vi "MAIN_TUBES_ANGGUN.vi"() -> ()   [LabVIEW 2025]
uses:
  <vilib>/addons/database/Connection.llb/DB Tools Open Connec (Path).vi
  <vilib>/Instr/_visa.llb/VISA Configure Serial Port (Instr).vi
  <vilib>/addons/database/Auxilliary.llb/DB Tools Format Datetime String (Time Stamp).vi
  <vilib>/addons/database/NI_Database_API.lvlib
panel:
  out "Time Stamp Indicator - Tall 5":timestamp format="%<%.0X\n%x>T"
  out "concatenated string":string
  out "Hasil Query 3":string
  out "error out 6":errorcluster
  out "Hasil Query 2":string
  out "concatenated string 2":string
  out "DatabaseSensor":bool
  out "error out 5":errorcluster
  in  "error in":errorcluster
  out "Ultra":string
  out "error out 4":errorcluster
  out "element":string
  out "Numeric":i32
  out "x+y":i32
  out "index of element":i32
  out "s? t:f":i32
  out "output array":string[](array[string])
  out "Array identitas":string[][](array[string])
  out "status Sistem":bool
  out "Hasil Query":string
  in  "error in (no error) 6":errorcluster
  out "error in (no error) 5":errorcluster
  out "Datetime":string
  in  "baud rate (9600)":u32=115200
  out "Com":string
  out "Pressure":string
  out "Suhu":string
  out "Serial Settings:Number of Bytes at Serial Port":u32
  out "Kemiringan":string
  out "Relay":string
  out "Motor":string
  in  "Tab Control 2":enum32{"Page 1"}(tab)
  out "Cancel":bool
  out "error out 2":errorcluster
  out "Hardware and Database":bool
  out "Login by":string
  out "Cancel 2":bool
  out "error out 3":errorcluster
  in  "error in (no error)":errorcluster
  in  "error in (no error) 2":errorcluster
  in  "error in (no error) 3":errorcluster
  out "Array tables":string[][](array[string])
  in  "error in (no error) 4":errorcluster
  out "error out":errorcluster
  in  "Tab Control":T1(tab)
  out "Role":string
  out "Time Stamp Indicator - Tall":timestamp format="%<%.0X\n%x>T"
  in  "Database":bool
  in  "Sign Up":bool
  in  "Log Out Square":bool
  in  "Graph Button":bool
  out "SERVO":bool
  out "POMPA":bool
  out "GRAFIK SENSOR ULTRASONIC":waveform(dbl)(graph) caption="Waveform Chart - Dark"
  out "MOTOR 2":bool
  out "INFRARED 2":bool
  out "MAX":bool
  out "MIN":bool
  out "WATER LEVEL TANK 2":dbl(slide) scale=0.0..10.0
  out "Time Stamp Indicator - Tall 3":timestamp format="%<%.0X\n%x>T"
  in  "Tab Setting":enum32{"Page 1"}(tab)
  out "read buffer":string
  in  "Nilai":string(combo)
  in  "Pilihan Sensor & Aktuator":string(combo)
  in  "Settings Button":bool
  in  "write buffer":string
  in  "Delay":string
  in  "Database  2":bool
  in  "Home Button":bool
  out "Pompa":string
  out "Motor 2":string
  out "Infra":string
  out "GRAFIK SENSOR INFRARED":waveform(i32)(graph) caption="Waveform Chart - Dark"
  out "Servo":string
  in  "Refresh Square":bool
  in  "Combo Box - Autocomplete":string(combo)
  in  "Combo Box - Dropdown 2":string(combo)
  in  "Search Button":bool
  in  "Database Sensor":bool
  in  "TABEL DATA USER":i32(listbox)
  in  "Home Button 2":bool
  in  "Graph Button 2":bool
  in  "connection information":path=path "D:/TUBES_SCADA_FIX/database.udl"
  out "Time Stamp Indicator - Tall 2":timestamp format="%<%.0X\n%x>T"
  in  "ATUR WAKTU":timestamp format="%<%.0X %x>T"
  in  "Combo Box - Dropdown 3":string(combo)
  in  "Combo Box - Autocomplete 2":string(combo)
  in  "Refresh Square 2":bool
  in  "Search Button 2":bool
  out "Time Stamp Indicator - Tall 4":timestamp format="%<%.0X\n%x>T"
  in  "Database User":bool
  in  "TABEL DATA SENSOR":i32(listbox)
  in  "Home Button 3":bool
  in  "Graph Button 3":bool
  # "(231, 230, 230)"
  # "RANCANG BANGUN MONITORING  FILLING MACHINE WITH LABVIEW"
  # "GRAFIK SENSOR ULTRASONIC"
  # "CM"
  # "GRAFIK SENSOR INFRARED"
  # "Jumlah Pembacaan Sensor &"
  # "Aksi Aktuator (Hidup/Mati)"
  # "Waktu Delay Setiap Pembacaan"
  # "MENCARI DATA USER"
  # "Refresh"
  # "MENCARI DATA SENSOR"
  # "Refresh"
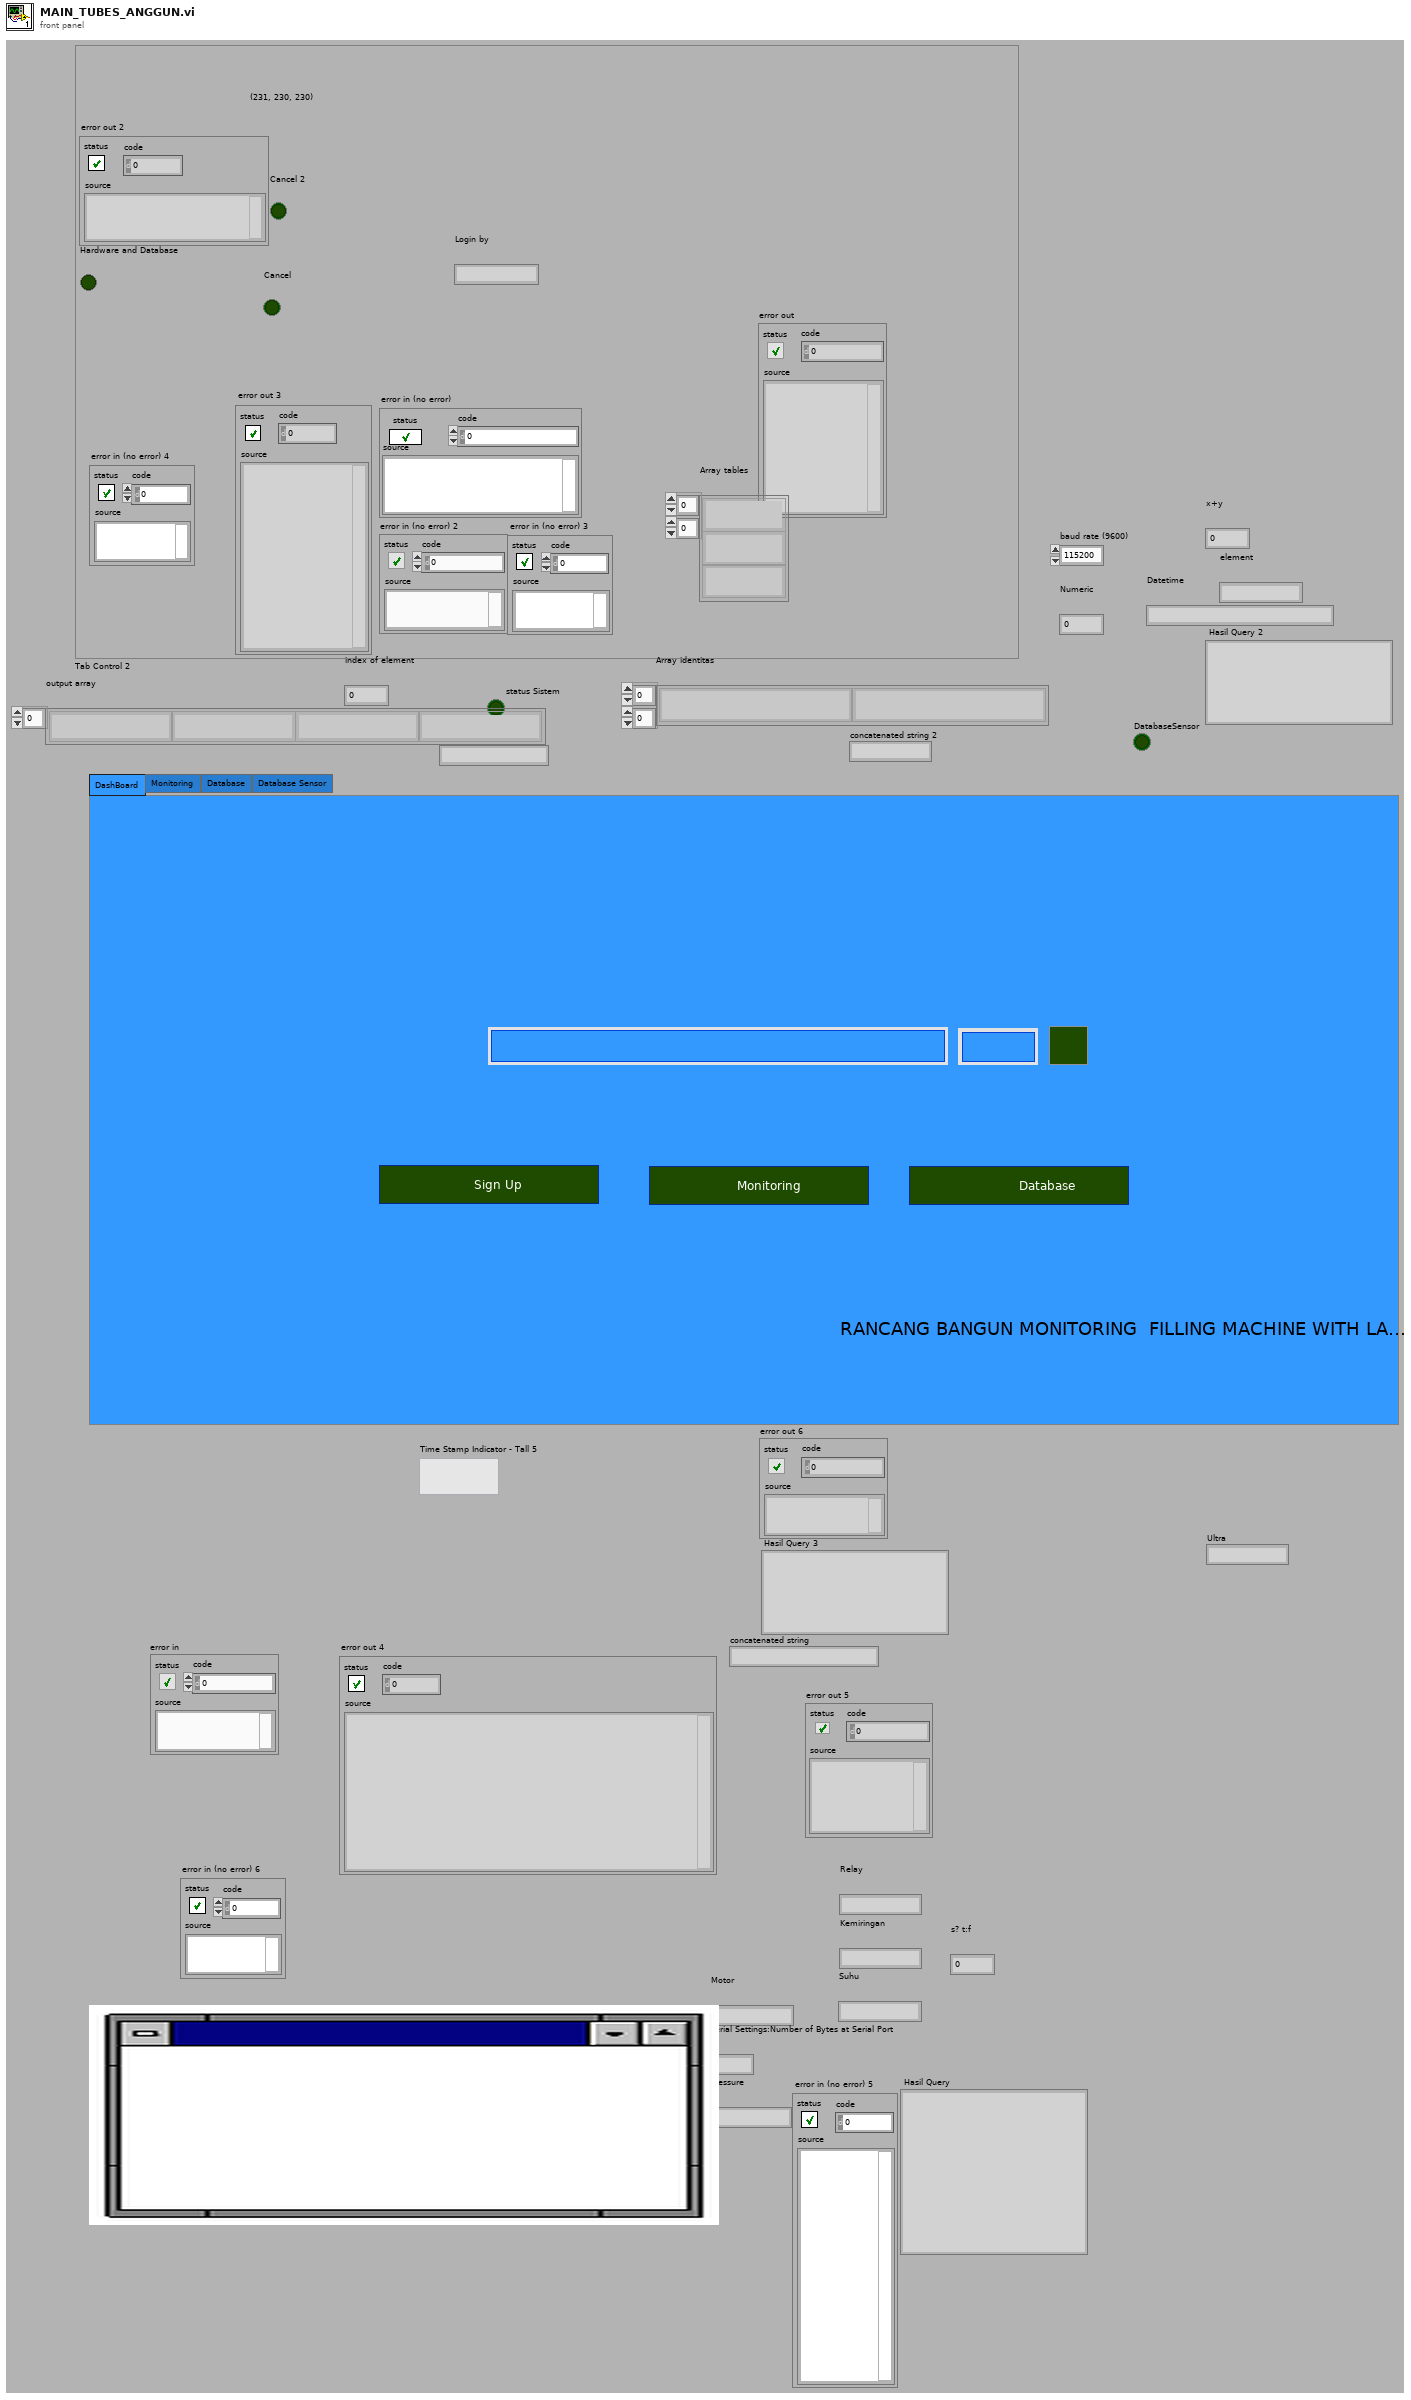
[diagram p1: front panel]
types:
  T1 = enum32{"DashBoard", "Monitoring", "Database", "Database Sensor"}
  T2 = typedef "NI_Database_API.lvlib/Conn ObjectReference.ctl" = refnum<k1>
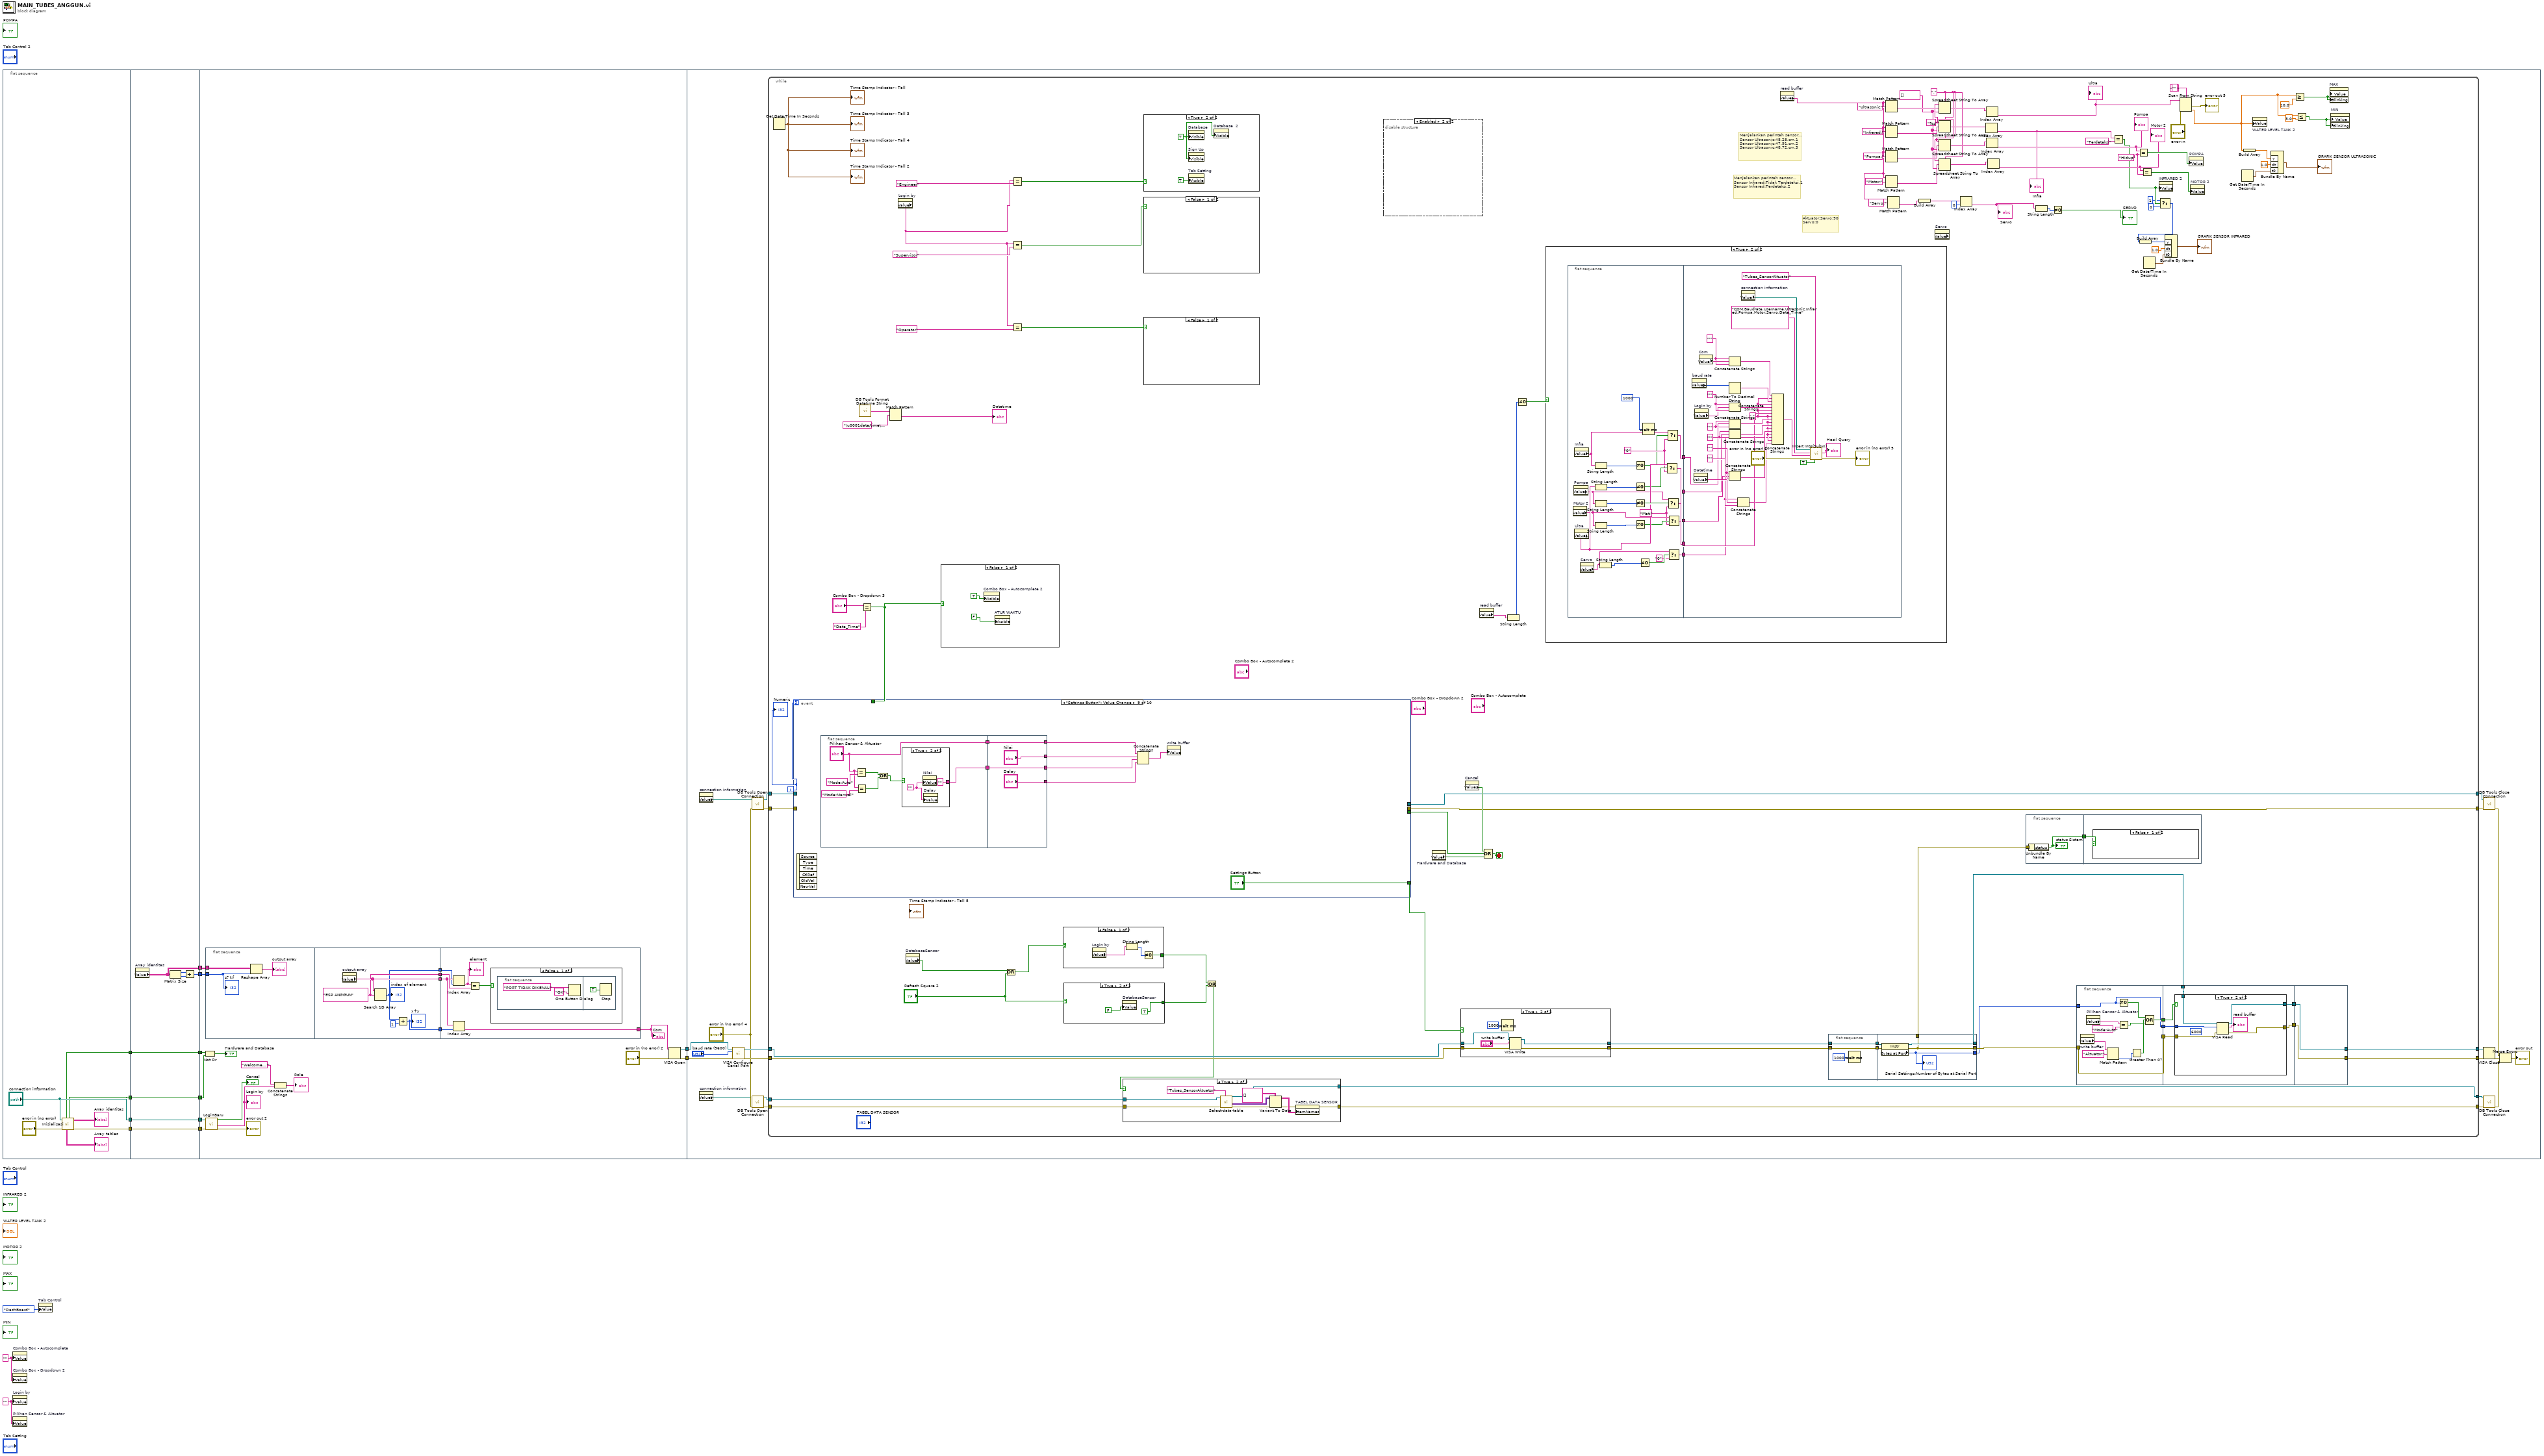
[diagram p0: block diagram]
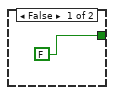
[diagram p3: hidden frame]
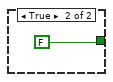
[diagram p4: hidden frame]
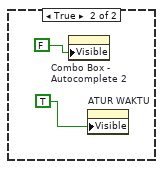
[diagram p5: hidden frame]
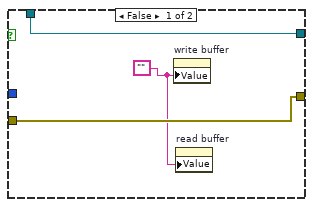
[diagram p6: hidden frame]
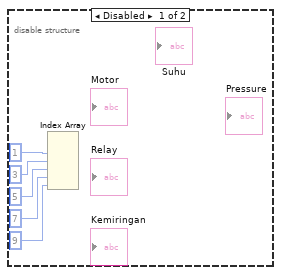
[diagram p7: hidden frame]
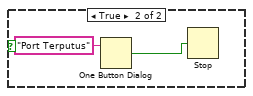
[diagram p8: hidden frame]
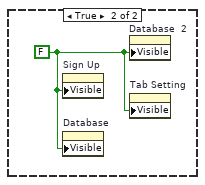
[diagram p11: hidden frame]
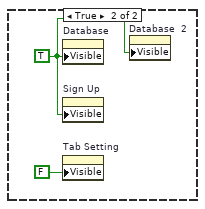
[diagram p12: hidden frame]
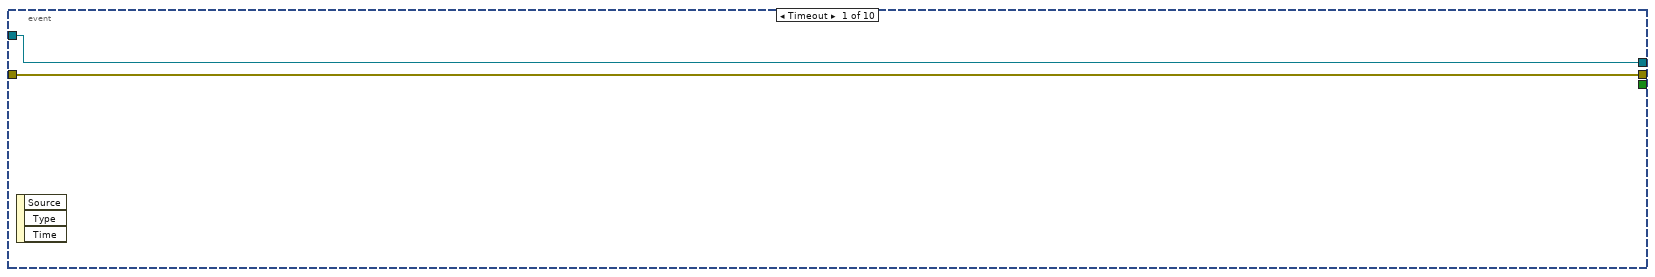
[diagram p15: hidden frame]
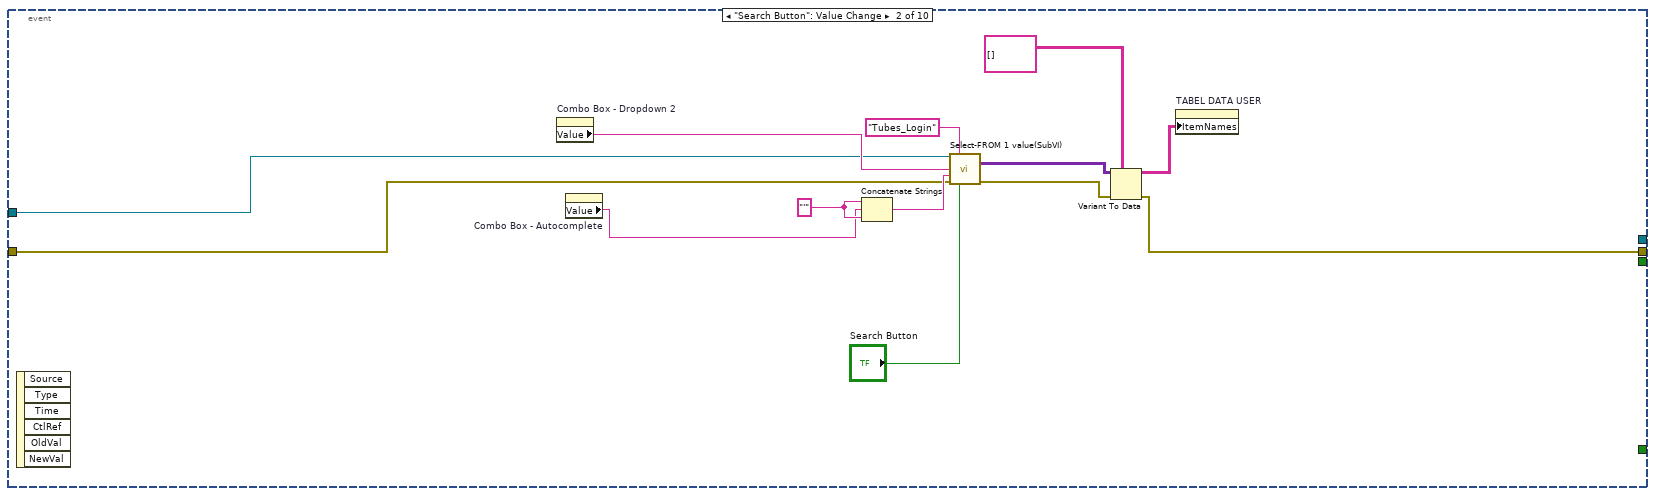
[diagram p16: hidden frame]
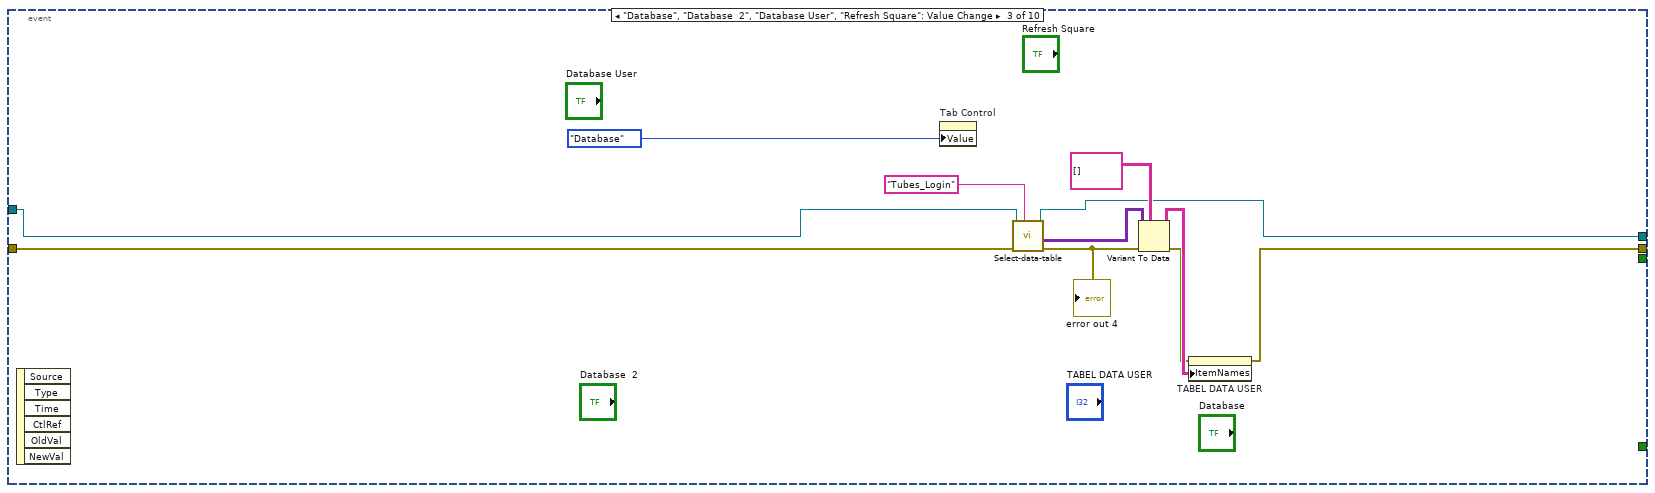
[diagram p17: hidden frame]
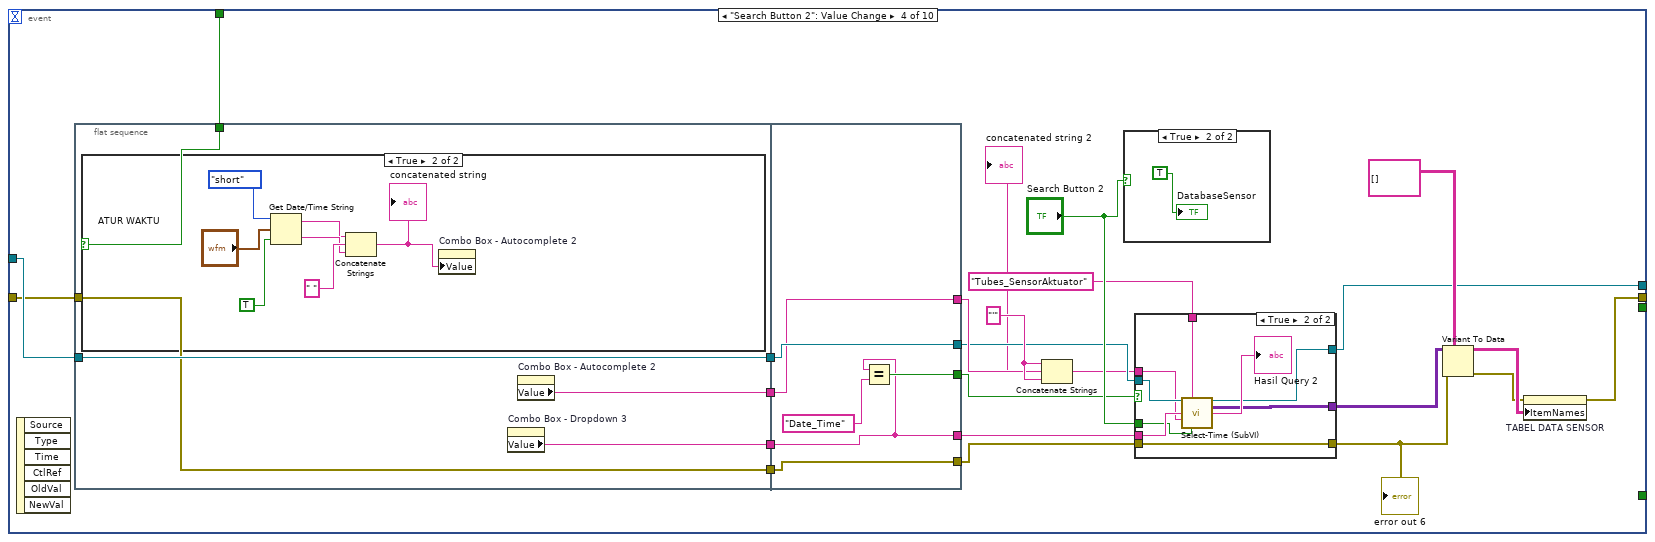
[diagram p18: hidden frame]
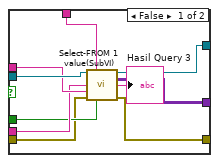
[diagram p19: hidden frame]
diagram:
  w1 = ""
  w2 = ""
  n1 = flat-sequence {
    tunnel: [w21] -> w12
    tunnel: ["connection information"] -> w10
    tunnel: [w19] -> w8
    tunnel: [w18] -> w6
    tunnel: w12 -> [w30]
    tunnel: [w30] -> w11
    tunnel: w10 -> [w29]
    tunnel: [w29] -> w9
    tunnel: w8 -> [w28]
    tunnel: [w28] -> w7
    tunnel: w6 -> [w27]
    tunnel: [w27] -> w5
    tunnel: [w26] -> w4
    tunnel: [w23] -> w3
    tunnel: w11 -> [w50]
    tunnel: w9 -> [w49]
    tunnel: [w44] -> w15
    tunnel: [w43] -> w14
    tunnel: w7 -> [w41]
    tunnel: w5 -> [w40]
    tunnel: w4 -> [w35]
    tunnel: w3 -> [w31]
    tunnel: w15 -> [w90]
    tunnel: w14 -> [w89]
    frame #0 {
      n2 = call "Inisialisasi.vi"("error in (no error)"="error in (no error)", "connection information"="connection information") -> ("error out"=w21:errorcluster, "Array identitas"=→"Array identitas":string[][], "HARDWARE"=w19:bool, "Array tables"=→"Array tables":string[][], "DATABASE"=w18:bool)  [unwired: 3 in, 2 out]
    }
    frame #1 {
      n3 = property on="Array identitas" class="Arr (strict)"() -> ("Value"=w26:string[][])  [unwired: 2 in, 2 out]
      n4 = Matrix Size(0:w26) -> (1:w25:i32, 2:w24:i32)
      n5 = Add(x=w25, y=w24) -> (x+y=w23:i32)
    }
    frame #2 {
      n6 = Not Or(1:w41, 2:w40) -> (0:→"Hardware and Database":bool)
      n7 = flat-sequence {
        tunnel: w35 -> [w52]
        tunnel: w31 -> [w51]
        tunnel: [w57] -> w37
        tunnel: [w56] -> w36
        tunnel: [w55] -> w33
        tunnel: [w54] -> w32
        tunnel: [w63] -> w34
        tunnel: w37 -> [w65]
        tunnel: w36 -> [w62]
        tunnel: w33 -> [w64]
        tunnel: w32 -> [w61]
        frame #0 {
          n8 = Reshape Array(w52, w51) -> (→"output array":string[])
          "s? t:f" <- w51
        }
        frame #1 {
          w55 = "ESP ANGGUN" ("element")
          n9 = property on="output array" class="Arr (strict)"() -> ("Value"=w56:string[])  [unwired: 2 in, 2 out]
          n10 = Search 1D Array(1D array=w56, element=w55) -> (index of element=w54:i32)  [unwired: 1 in]
          "index of element" <- w54
          n11 = Add(x=w54, y=1 ("x")) -> (x+y=w57:i32)
          "x+y" <- w57
        }
        frame #2 {
          n12 = Index Array(array=w62, index=w61) -> (element=w60:string)
          "element" <- w60
          n13 = Index Array(array=w62, index=w65) -> (element=w63:string)
          n14 = Equal?(x=w60, y=w64) -> (x = y?=w59:bool)
          n15 = case shown="False" w59 {
            frame False {
              n16 = flat-sequence {
                frame #0 {
                  n17 = One Button Dialog(message="PORT TIDAK DIKENAL!", button name ("OK")="OK") -> ()  [unwired: 1 out]
                }
                frame #1 {
                  n18 = Stop(stop? (T)=TRUE) -> ()
                }
              }
            }
            frame True {
            }
          }
        }
      }
      n19 = call "LoginBaru.vi"("error in (no error)"=w50, "connection information"=w49) -> ("error out 2"=→"error out 2":errorcluster, "Role"=w47:string, "Cancel"=→"Cancel":bool)  [unwired: 7 in]
      "Login by" <- w47
      n20 = Concatenate Strings("Welcome...!" ("string"), w47) -> (→"Role":string)
      n21 = VISA Open(error in (no error)="error in (no error) 2", VISA resource name=w34) -> (VISA resource name=w44:refnum<visa-resource-name>, error out=w43:errorcluster)  [unwired: 3 in]
      "Com" <- w34
    }
    frame #3 {
      n22 = property on="connection information" class="Path"() -> ("Value"=w84:path)  [unwired: 2 in, 2 out]
      n23 = property on="connection information" class="Path"() -> ("Value"=w71:path)  [unwired: 2 in, 2 out]
      n24 = call-poly "VISA Configure Serial Port"("VISA resource name"=w90, "baud rate (9600)"="baud rate (9600)", "error in (no error)"=w89) -> ("VISA resource name out"=w88:refnum<visa-resource-name>, "error out"=w87:errorcluster)  [unwired: 11 in]
      n25 = call-poly <vilib>:"DB Tools Open Connection.vi"("error in (no error)"="error in (no error) 4", "connection information"=w84) -> ("error out"=w83:errorcluster, "connection reference"=w85:T2)  [unwired: 6 in]
      n26 = call-poly <vilib>:"DB Tools Open Connection.vi"("error in (no error)"="error in (no error) 4", "connection information"=w71) -> ("error out"=w73:errorcluster, "connection reference"=w72:T2)  [unwired: 6 in]
      n27 = while {
        tunnel: w88 -> [w195]
        tunnel: w87 -> [w170]
        tunnel: w85 -> [w179]
        tunnel: w83 -> [w178]
        tunnel: [w177] -> w82
        tunnel: w73 -> [w176]
        tunnel: [w175] -> w76
        tunnel: [w164] -> w78
        tunnel: [w162] -> w75
        tunnel: w72 -> [w161]
        tunnel: [w153] -> w70
        tunnel: [w152] -> w69
        i -> [w196]
        stop <- w188 stop-if-true
        w129 = "Hidup" ("y")
        (unwired) "%f" ("format string")
        w141 = "," ("delimiter (Tab)")
        w142 = "%s" ("format string")
        w143 = string[] []
        # "Aktuator:Servo:90\nServo:0"
        # "Menjalankan perintah sensor...\nSensor Infrared:Tidak Terdeteksi,1\nSensor Infrared:Terdeteksi,2"
        # "Menjalankan perintah sensor...\nSensor Ultrasonic:48.28,cm,1\nSensor Ultrasonic:47.91,cm,2\nSensor Ultrasonic:48.72,cm,3"
        n28 = Get Date/Time In Seconds() -> (seconds since 1Jan1904=→"Time Stamp Indicator - Tall" →"Time Stamp Indicator - Tall 3" →"Time Stamp Indicator - Tall 4" →"Time Stamp Indicator - Tall 2":timestamp)
        n29 = call-poly <vilib>:"DB Tools Format Datetime String.vi"() -> ("date/time string"=w173:string)  [unwired: 1 in]
        n30 = Equal?(x="Combo Box - Dropdown 3", y="Date_Time" ("Combo Box - Dropdown 3")) -> (x = y?=w106:bool)
        n31 = event shown="[8] \"Settings Button\": Value Change" {
          selector: _ -> [_ _ _ _ _ _ _ _ _ _]
          dyn-events: _ -> [_ _ _ _ _ _ _ _ _ _]
          timeout: w196 -> [_ _ _ _ _ _ _ _ _ _]
          tunnel: [w339 _ w355 w366 _ _ _ _ _ _] -> w164
          tunnel: [_ _ _ _ _ _ _ _ "Settings Button" _] -> w187
          tunnel: w179 -> [w339 w348 w354 w386 _ _ _ _ _ _]
          tunnel: w178 -> [w340 w347 w363 w384 _ _ _ _ _ _]
          tunnel: [w340 w345 w357 w367 _ _ _ _ _ _] -> w177
          tunnel: [_ _ _ _ _ _ _ _ _ w456] -> w163
          tunnel: w106 -> [_ _ _ w365 _ _ _ _ _ _]
          event Timeout {
            n32 = event-data() -> ()  [unwired: 1 in, 3 out]
          }
          event "Search Button": Value Change {
            w352 = "'"
            n33 = event-data() -> ()  [unwired: 1 in, 6 out]
            n34 = property on="Combo Box - Dropdown 2" class="CmbBox"() -> ("Value"=w349:string)  [unwired: 2 in, 2 out]
            n35 = property on="Combo Box - Autocomplete" class="CmbBox"() -> ("Value"=w351:string)  [unwired: 2 in, 2 out]
            n36 = Concatenate Strings(w352, w351, w352) -> (w350:string)
            n37 = call "Select-FROM 1 value(SubVI).vi"("connection reference"=w348, "TABLE"="Tubes_Login", "COLOUM Data"=w349, "Nilainya"=w350, "error in (no error)"=w347, "Cari"="Search Button") -> ("recordset data"=w343:variant[][], "error out"=w346:errorcluster)  [unwired: 5 in, 3 out]
            n38 = Variant To Data(error in=w346, type=string[][] [], Variant=w343) -> (data=w342:string[][], error out=w345:errorcluster)
            n39 = property on="TABEL DATA USER" class="MCListbox (strict)"("ItemNames"=w342) -> ()  [unwired: 2 in, 2 out]
          }
          event "Database", "Database  2", "Database User", "Refresh Square": Value Change {
            n40 = event-data() -> ()  [unwired: 1 in, 6 out]
            n41 = property on="Tab Control" class="TabCtl (strict)"("Value"=enum32{"DashBoard", "Monitoring", "Database"}."Database" ("Tab Control")) -> ()  [unwired: 2 in, 2 out]
            n42 = call "Select-data-table.vi"("TABLE NAME"="Tubes_Login", "error in (no error)"=w363, "connection reference"=w354) -> ("error out"=w361:errorcluster, "recordset data"=w356:variant[][], "connection reference 2"=w355:T2)  [unwired: 5 in, 1 out]
            "error out 4" <- w361
            n43 = Variant To Data(error in=w361, type=string[][] [] ("Item Names"), Variant=w356) -> (data=w359:string[][], error out=w358:errorcluster)
            n44 = property on="TABEL DATA USER" class="MCListbox (strict)"(error in=w358, "ItemNames"=w359) -> (error out=w357:errorcluster)  [unwired: 1 in, 1 out]
          }
          event "Search Button 2": Value Change {
            w381 = "'"
            n45 = event-data() -> ()  [unwired: 1 in, 6 out]
            n46 = flat-sequence {
              tunnel: [w412] -> w387
              tunnel: w386 -> [w412]
              tunnel: [w411] -> w385
              tunnel: w384 -> [w411]
              tunnel: [w410] -> w383
              tunnel: [w409] -> w382
              tunnel: w365 -> [w408]
              tunnel: w387 -> [w422]
              tunnel: w385 -> [w424]
              tunnel: w383 -> [w420]
              tunnel: [w424] -> w370
              tunnel: [w423] -> w377
              tunnel: [w422] -> w378
              tunnel: [w421] -> w380
              tunnel: w382 -> [w421]
              tunnel: [w420] -> w375
              frame #0 {
                n47 = case shown="True" w408 {
                  frame False {
                  }
                  frame True {
                    n48 = Get Date/Time String(date format (0)=enum16{"short", "long", "abbreviated"}."short", seconds (now)="ATUR WAKTU", want seconds? (F)=TRUE) -> (date string=w417:string, time string=w418:string)
                    n49 = Concatenate Strings(w417, " ", w418) -> (w415:string)
                    "concatenated string" <- w415
                    n50 = property on="Combo Box - Autocomplete 2" class="CmbBox"("Value"=w415) -> ()  [unwired: 2 in, 2 out]
                  }
                }
                n51 = property on="Combo Box - Dropdown 3" class="CmbBox"() -> ("Value"=w410:string)  [unwired: 2 in, 2 out]
                n52 = property on="Combo Box - Autocomplete 2" class="CmbBox"() -> ("Value"=w409:string)  [unwired: 2 in, 2 out]
              }
              frame #1 {
                n53 = Equal?(x=w420, y="Date_Time" ("Combo Box - Dropdown 3")) -> (x = y?=w423:bool)
              }
            }
            n54 = Concatenate Strings(w381, w380, w381) -> (w374:string)
            "concatenated string 2" <- w374
            n55 = case shown="True" "Search Button 2" {
              frame False {
              }
              frame True {
                "DatabaseSensor" <- TRUE
              }
            }
            n56 = case shown="True" w377 {
              tunnel: "Search Button 2" -> [w393 w402]
              tunnel: w378 -> [w397 w405]
              tunnel: "Tubes_SensorAktuator" ("TABLE") -> [w396 w406]
              tunnel: w375 -> [w394 w404]
              tunnel: w374 -> [w395 w403]
              tunnel: [w392 w400] -> w371
              tunnel: w370 -> [w390 w399]
              tunnel: [w391 w399] -> w369
              tunnel: [w389 w398] -> w366
              frame False {
                n57 = call "Select-FROM 1 value(SubVI).vi"("connection reference"=w397, "TABLE"=w396, "COLOUM Data"=w394, "Nilainya"=w395, "error in (no error)"=w390, "Cari"=w393) -> ("connection reference 2"=w389:T2, "recordset data"=w392:variant[][], "Hasil Query"=→"Hasil Query 3":string, "error out"=w391:errorcluster)  [unwired: 5 in, 1 out]
              }
              frame True {
                n58 = call "Select-Time (SubVI).vi"("connection reference"=w405, "TABLE"=w406, "COLOUM Date_Time"=w404, "Nilainya"=w403, "Cari"=w402) -> ("connection reference 2"=w398:T2, "recordset data"=w400:variant[][], "Hasil Query"=→"Hasil Query 2":string)  [unwired: 6 in, 2 out]
              }
            }
            "error out 6" <- w369
            n59 = Variant To Data(error in=w369, type=string[][] [], Variant=w371) -> (data=w372:string[][], error out=w368:errorcluster)
            n60 = property on="TABEL DATA SENSOR" class="MCListbox (strict)"(error in=w368, "ItemNames"=w372) -> (error out=w367:errorcluster)  [unwired: 1 in, 1 out]
          }
          event "Database Sensor": Value Change {
            n61 = event-data() -> ()  [unwired: 1 in, 6 out]
            n62 = property on="Tab Control" class="TabCtl (strict)"("Value"=T1."Database Sensor" ("Tab Control")) -> ()  [unwired: 2 in, 2 out]
          }
          event "Sign Up": Value Change {
            n63 = event-data() -> ()  [unwired: 1 in, 6 out]
            n64 = property on="connection information" class="Path"() -> ("Value"=w431:path)  [unwired: 2 in, 2 out]
            n65 = property on="Login by" class="Str"() -> ("Value"=w428:string)  [unwired: 2 in, 2 out]
            n66 = call "Sign in tubes.vi"("error in (no error)"="error in (no error) 3", "Create By"=w428, "connection information"=w431) -> ("error out"=→"error out 3":errorcluster, "Cancel"=→"Cancel 2":bool)  [unwired: 7 in]
          }
          event "Graph Button 3", "Graph Button 2", "Graph Button": Value Change {
            n67 = event-data() -> ()  [unwired: 1 in, 6 out]
            n68 = property on="Tab Control" class="TabCtl (strict)"("Value"=enum32{"DashBoard", "Monitoring", "Database"}."Monitoring" ("Tab Control")) -> ()  [unwired: 2 in, 2 out]
          }
          event "Home Button", "Home Button 2", "Home Button 3": Value Change {
            n69 = event-data() -> ()  [unwired: 1 in, 6 out]
            n70 = property on="Tab Control" class="TabCtl (strict)"("Value"=enum32{"DashBoard", "Monitoring", "Database"}."DashBoard" ("Tab Control")) -> ()  [unwired: 2 in, 2 out]
          }
          event "Settings Button": Value Change {
            n71 = event-data() -> ()  [unwired: 1 in, 6 out]
            n72 = flat-sequence {
              tunnel: [w443] -> w436
              tunnel: ["Pilihan Sensor & Aktuator"] -> w434
              tunnel: ["Nilai"] -> w439
              tunnel: ["Delay"] -> w438
              tunnel: [w453] -> w437
              tunnel: w436 -> [w453]
              tunnel: [w452] -> w435
              tunnel: w434 -> [w452]
              frame #0 {
                n73 = Equal?(x="Pilihan Sensor & Aktuator", y="Mode:Auto" ("Type")) -> (x = y?=w446:bool)
                n74 = Equal?(x="Pilihan Sensor & Aktuator", y="Mode:Manual" ("Type")) -> (x = y?=w445:bool)
                n75 = Or(x=w446, y=w445) -> (x .or. y?=w444:bool)
                n76 = case shown="True" w444 {
                  tunnel: [":" ("string") "" ("string")] -> w443
                  frame False {
                  }
                  frame True {
                    w451 = ""
                    n77 = property on="Nilai" class="CmbBox"("Value"=w451) -> ()  [unwired: 2 in, 2 out]
                    n78 = property on="Delay" class="Str"("Value"=w451) -> ()  [unwired: 2 in, 2 out]
                  }
                }
              }
              frame #1 {
              }
            }
            n79 = Concatenate Strings(w435, w439, w437, w438) -> (w441:string)
            n80 = property on="write buffer" class="Str"("Value"=w441) -> ()  [unwired: 2 in, 2 out]
          }
          event "Log Out Square": Value Change {
            n81 = event-data() -> ()  [unwired: 1 in, 6 out]
            n82 = Two Button Dialog(message="Apa Anda Yakin Ingin Keluar?", 1:"TIDAK" ("F button name (\"Cancel\")"), 2:"YA" ("T button name (\"OK\")")) -> (T button?=w456:bool)
          }
        }
        n83 = Match Pattern(string=w173, regular expression="\u0001date/time\u0001") -> (after substring=→"Datetime":string)  [unwired: 1 in, 3 out]
        n84 = property on="Login by" class="Str"() -> ("Value"=w180:string)  [unwired: 2 in, 2 out]
        n85 = property on="DatabaseSensor" class="Bool (strict)"() -> ("Value"=w105:bool)  [unwired: 2 in, 2 out]
        n86 = case shown="False" w106 {
          frame False {
            n87 = property on="Combo Box - Autocomplete 2" class="CmbBox"("Visible"=TRUE) -> ()  [unwired: 2 in, 2 out]
            n88 = property on="ATUR WAKTU" class="AbsTime (strict)"("Visible"=FALSE) -> ()  [unwired: 2 in, 2 out]
          }
          frame True {
            n89 = property on="Combo Box - Autocomplete 2" class="CmbBox"("Visible"=FALSE) -> ()  [unwired: 2 in, 2 out]
            n90 = property on="ATUR WAKTU" class="AbsTime (strict)"("Visible"=TRUE) -> ()  [unwired: 2 in, 2 out]
          }
        }
        n91 = Or(x=w105, y="Refresh Square 2") -> (x .or. y?=w104:bool)
        n92 = Equal?(x=w180, y="Engineer") -> (x = y?=w185:bool)
        n93 = Equal?(x=w180, y="Supervisor") -> (x = y?=w183:bool)
        n94 = Equal?(x=w180, y="Operator") -> (x = y?=w181:bool)
        n95 = case shown="False" w104 {
          tunnel: [w200 FALSE] -> w103
          frame False {
            n96 = property on="Login by" class="Str"() -> ("Value"=w202:string)  [unwired: 2 in, 2 out]
            n97 = String Length(string=w202) -> (length=w201:i32)
            n98 = Not Equal To 0?(x=w201) -> (x != 0?=w200:bool)
          }
          frame True {
          }
        }
        n99 = case shown="True" "Refresh Square 2" {
          tunnel: [FALSE TRUE] -> w100
          frame False {
          }
          frame True {
            n100 = property on="DatabaseSensor" class="Bool (strict)"("Value"=FALSE) -> ()  [unwired: 2 in, 2 out]
          }
        }
        n101 = case shown="True" w185 {
          frame False {
          }
          frame True {
            w321 = TRUE ("Visible")
            n102 = property on="Database" class="Bool"("Visible"=w321) -> ()  [unwired: 2 in, 2 out]
            n103 = property on="Sign Up" class="Bool"("Visible"=w321) -> ()  [unwired: 2 in, 2 out]
            n104 = property on="Tab Setting" class="TabCtl (strict)"("Visible"=TRUE) -> ()  [unwired: 2 in, 2 out]
            n105 = property on="Database  2" class="Bool"("Visible"=w321) -> ()  [unwired: 2 in, 2 out]
          }
        }
        n106 = case shown="False" w183 {
          frame False {
          }
          frame True {
            w319 = TRUE ("Visible")
            n107 = property on="Database" class="Bool"("Visible"=w319) -> ()  [unwired: 2 in, 2 out]
            n108 = property on="Sign Up" class="Bool"("Visible"=w319) -> ()  [unwired: 2 in, 2 out]
            n109 = property on="Tab Setting" class="TabCtl (strict)"("Visible"=FALSE) -> ()  [unwired: 2 in, 2 out]
            n110 = property on="Database  2" class="Bool"("Visible"=w319) -> ()  [unwired: 2 in, 2 out]
          }
        }
        n111 = case shown="False" w181 {
          frame False {
          }
          frame True {
            w318 = FALSE ("Visible")
            n112 = property on="Sign Up" class="Bool"("Visible"=w318) -> ()  [unwired: 2 in, 2 out]
            n113 = property on="Database" class="Bool"("Visible"=w318) -> ()  [unwired: 2 in, 2 out]
            n114 = property on="Database  2" class="Bool"("Visible"=w318) -> ()  [unwired: 2 in, 2 out]
            n115 = property on="Tab Setting" class="TabCtl (strict)"("Visible"=w318) -> ()  [unwired: 2 in, 2 out]
          }
        }
        n116 = Or(x=w103, y=w100) -> (x .or. y?=w101:bool)
        n117 = case shown="True" w101 {
          tunnel: w176 -> [w307 w317]
          tunnel: [w307 w311] -> w175
          tunnel: [w306 w310] -> w162
          tunnel: w161 -> [w306 w309]
          frame False {
          }
          frame True {
            n118 = call "Select-data-table.vi"("TABLE NAME"="Tubes_SensorAktuator", "error in (no error)"=w317, "connection reference"=w309) -> ("error out"=w313:errorcluster, "recordset data"=w308:variant[][], "connection reference 2"=w310:T2)  [unwired: 5 in, 1 out]
            n119 = Variant To Data(error in=w313, type=string[][] [] ("Item Names"), Variant=w308) -> (data=w314:string[][], error out=w312:errorcluster)
            n120 = property on="TABEL DATA SENSOR" class="MCListbox (strict)"(error in=w312, "ItemNames"=w314) -> (error out=w311:errorcluster)  [unwired: 1 in, 1 out]
          }
        }
        n121 = disable-structure shown="Enabled" {
          frame Disabled {
            n122 = Index Array(index #1=1 ("index"), index #2=3 ("index"), index #3=5 ("index"), index #4=7 ("index"), index #5=9 ("index")) -> ()  [unwired: 1 in, 5 out]
          }
          frame Enabled {
          }
        }
        n123 = property on="Hardware and Database" class="Bool (strict)"() -> ("Value"=w189:bool)  [unwired: 2 in, 2 out]
        n124 = case shown="True" w187 {
          tunnel: w195 -> [w324 w330]
          tunnel: w170 -> [w323 w329]
          tunnel: [w324 w328] -> w194
          tunnel: [w323 w327] -> w193
          frame False {
          }
          frame True {
            n125 = Wait (ms)(milliseconds to wait=u32 1000) -> ()  [unwired: 1 out]
            n126 = VISA Write(VISA resource name=w330, write buffer="write buffer", error in (no error)=w329) -> (VISA resource name out=w328:refnum<visa-resource-name>, error out=w327:errorcluster)  [unwired: 1 out]
          }
        }
        n127 = property on="Cancel" class="Bool (strict)"() -> ("Value"=w190:bool)  [unwired: 2 in, 2 out]
        n128 = property on="read buffer" class="Str"() -> ("Value"=w167:string)  [unwired: 2 in, 2 out]
        n129 = Compound Arithmetic op=OR(w190, w163, w189) -> (w188:bool)
        n130 = String Length(string=w167) -> (length=w166:i32)
        n131 = Not Equal To 0?(x=w166) -> (x != 0?=w165:bool)
        n132 = case shown="True" w165 {
          frame False {
          }
          frame True {
            n133 = flat-sequence {
              tunnel: [w259] -> w250
              tunnel: [w258] -> w249
              tunnel: [w257] -> w248
              tunnel: [w256] -> w247
              tunnel: [w251] -> w246
              tunnel: w250 -> [w281]
              tunnel: w249 -> [w280]
              tunnel: w248 -> [w279]
              tunnel: w247 -> [w278]
              tunnel: w246 -> [w276]
              frame #0 {
                w260 = "Mati"
                w265 = "0"
                n134 = property on="Motor 2" class="Str"() -> ("Value"=w262:string)  [unwired: 2 in, 2 out]
                n135 = property on="Pompa" class="Str"() -> ("Value"=w263:string)  [unwired: 2 in, 2 out]
                n136 = property on="Infra" class="Str"() -> ("Value"=w266:string)  [unwired: 2 in, 2 out]
                n137 = property on="Ultra" class="Str"() -> ("Value"=w268:string)  [unwired: 2 in, 2 out]
                n138 = property on="Servo" class="Str"() -> ("Value"=w253:string)  [unwired: 2 in, 2 out]
                n139 = String Length(string=w266) -> (length=w272:i32)
                n140 = String Length(string=w268) -> (length=w273:i32)
                n141 = String Length(string=w263) -> (length=w271:i32)
                n142 = String Length(string=w262) -> (length=w270:i32)
                n143 = String Length(string=w253) -> (length=w255:i32)
                n144 = Not Equal To 0?(x=w272) -> (x != 0?=w264:bool)
                n145 = Not Equal To 0?(x=w273) -> (x != 0?=w267:bool)
                n146 = Not Equal To 0?(x=w271) -> (x != 0?=w269:bool)
                n147 = Not Equal To 0?(x=w270) -> (x != 0?=w261:bool)
                n148 = Not Equal To 0?(x=w255) -> (x != 0?=w254:bool)
                n149 = Wait (ms)(milliseconds to wait=u32 1000) -> ()  [unwired: 1 out]
                n150 = Select(t=w268, s=w267, f=w265) -> (s? t:f=w258:string)
                n151 = Select(t=w266, s=w264, f=w265) -> (s? t:f=w259:string)
                n152 = Select(t=w263, s=w269, f=w260) -> (s? t:f=w256:string)
                n153 = Select(t=w262, s=w261, f=w260) -> (s? t:f=w257:string)
                n154 = Select(t=w253, s=w254, f="0") -> (s? t:f=w251:string)
              }
              frame #1 {
                w282 = "'" ("string")
                w290 = "'" ("string")
                w293 = "'" ("string")
                w295 = "'" ("string")
                w297 = "'" ("string")
                w277 = "," ("string")
                w300 = "'" ("string")
                n155 = property on="baud rate" class="DigNum (strict)"() -> ("Value"=w305:u32)  [unwired: 2 in, 2 out]
                n156 = property on="Datetime" class="Str"() -> ("Value"=w291:string)  [unwired: 2 in, 2 out]
                n157 = property on="Login by" class="Str"() -> ("Value"=w285:string)  [unwired: 2 in, 2 out]
                n158 = property on="Com" class="Str"() -> ("Value"=w301:string)  [unwired: 2 in, 2 out]
                n159 = Concatenate Strings(w300, w301, w300) -> (w299:string)
                n160 = Number To Decimal String(number=w305) -> (decimal integer string=w298:string)  [unwired: 1 in]
                n161 = Concatenate Strings(w297, w285, w297) -> (w296:string)
                n162 = Concatenate Strings(w282, w281, w282) -> (w283:string)
                n163 = Concatenate Strings(w295, w278, w295) -> (w294:string)
                n164 = Concatenate Strings(w293, w279, w293) -> (w292:string)
                n165 = Concatenate Strings(w290, w291, w290) -> (w275:string)
                n166 = property on="connection information" class="Path"() -> ("Value"=w304:path)  [unwired: 2 in, 2 out]
                n167 = Concatenate Strings(w299, w277, w298, w277, w296, w277, w280, w277, w283, w277, w294, w277, w292, w277, w276, w277, w275) -> (w289:string)
                n168 = call "Insert Into(SubVI).vi"("Boolean"=TRUE, "TABLE NAME"="Tubes_SensorAktuator", "error in (no error)"="error in (no error) 6", "VALUE DATA"=w289, "COLUMN NAME"="COM,Baudrate,Username,Ultrasonic,Infrared,Pompa,Motor,Servo,Date_Time", "connection information"=w304) -> ("error out"=→"error in (no error) 5":errorcluster, "Hasil Query"=→"Hasil Query":string)  [unwired: 4 in]
              }
            }
          }
        }
        n169 = property on="read buffer" class="Str"() -> ("Value"=w99:string)  [unwired: 2 in, 2 out]
        n170 = flat-sequence {
          tunnel: w193 -> [w332]
          tunnel: w194 -> [w333]
          tunnel: [w333] -> w192
          tunnel: [w332] -> w191
          tunnel: [w336] -> w158
          tunnel: [w335] -> w157
          tunnel: w192 -> [w338]
          tunnel: w191 -> [w337]
          tunnel: [w335] -> w169
          tunnel: [w334] -> w155
          frame #0 {
            n171 = Wait (ms)(milliseconds to wait=u32 1000) -> ()  [unwired: 1 out]
          }
          frame #1 {
            n172 = property class="Instr"(reference=w338, error in=w337) -> (reference out=w336:refnum<visa-resource-name>, error out=w335:errorcluster, "Bytes at Port"=w334:u32)
            "Serial Settings:Number of Bytes at Serial Port" <- w334
          }
        }
        n173 = Match Pattern(string=w99, regular expression="Ultrasonic:") -> (after substring=w147:string)  [unwired: 1 in, 3 out]
        n174 = Match Pattern(string=w99, regular expression="Infrared:") -> (after substring=w146:string)  [unwired: 1 in, 3 out]
        n175 = Match Pattern(string=w99, regular expression="Pompa:") -> (after substring=w145:string)  [unwired: 1 in, 3 out]
        n176 = Match Pattern(string=w99, regular expression="Motor:") -> (after substring=w144:string)  [unwired: 1 in, 3 out]
        n177 = Match Pattern(string=w99, regular expression="Servo:") -> (after substring=w97:string)  [unwired: 1 in, 3 out]
        n178 = Build Array(w97) -> (w96:string[])
        n179 = property on="Servo" class="Str" props=["Value"]() -> ()  [unwired: 2 in, 3 out]
        n180 = Spreadsheet String To Array(delimiter (Tab)=w141, format string=w142, spreadsheet string=w147, array type (2D Dbl)=w143) -> (array=w140:string[])
        n181 = Spreadsheet String To Array(delimiter (Tab)=w141, format string=w142, spreadsheet string=w146, array type (2D Dbl)=w143) -> (array=w139:string[])
        n182 = Spreadsheet String To Array(delimiter (Tab)=w141, format string=w142, spreadsheet string=w145, array type (2D Dbl)=w143) -> (array=w138:string[])
        n183 = Spreadsheet String To Array(delimiter (Tab)=w141, format string=w142, spreadsheet string=w144, array type (2D Dbl)=w143) -> (array=w137:string[])
        n184 = Index Array(array=w96, index=0) -> (element=w94:string)
        "Servo" <- w94
        n185 = Index Array(array=w139) -> (element=w117:string)  [unwired: 1 in]
        "Infra" <- w117
        n186 = Index Array(array=w140) -> (element=w136:string)  [unwired: 1 in]
        "Ultra" <- w136
        n187 = Index Array(array=w138) -> (element=w132:string)  [unwired: 1 in]
        "Pompa" <- w132
        n188 = Index Array(array=w137) -> (element=w130:string)  [unwired: 1 in]
        "Motor 2" <- w130
        n189 = flat-sequence {
          tunnel: w169 -> [w242]
          tunnel: [w241] -> w168
          tunnel: w168 -> [w243]
          frame #0 {
            n190 = Unbundle By Name(w242) -> ("status"=w241:bool)
            "status Sistem" <- w241
          }
          frame #1 {
            n191 = case shown="False" w243 {
              frame False {
              }
              frame True {
                n192 = One Button Dialog(message="Port Terputus") -> (true=w244:bool)  [unwired: 1 in]
                n193 = Stop(stop? (T)=w244) -> ()
              }
            }
          }
        }
        n194 = String Length(string=w94) -> (length=w93:i32)
        n195 = Not Equal To 0?(x=w93) -> (x != 0?=→"SERVO":bool)
        n196 = flat-sequence {
          tunnel: w157 -> [w218]
          tunnel: [w218] -> w156
          tunnel: w155 -> [w208]
          tunnel: [w213] -> w154
          tunnel: [w208] -> w91
          tunnel: [w222] -> w160
          tunnel: [w223] -> w159
          tunnel: w158 -> [w224]
          tunnel: w156 -> [w221]
          tunnel: w154 -> [w220]
          tunnel: w91 -> [w219]
          tunnel: w160 -> [w234]
          tunnel: w159 -> [w235]
          tunnel: [w235] -> w153
          tunnel: [w234] -> w152
          frame #0 {
            n197 = property on="write buffer" class="Str"() -> ("Value"=w212:string)  [unwired: 2 in, 2 out]
            n198 = property on="Pilihan Sensor & Aktuator" class="CmbBox"() -> ("Value"=w211:string)  [unwired: 2 in, 2 out]
            n199 = Match Pattern(string=w212, regular expression="Aktuator:") -> (offset past match=w215:i32)  [unwired: 1 in, 3 out]
            n200 = Not Equal To 0?(x=w208) -> (x != 0?=w217:bool)
            n201 = Equal?(x=w211, y="Mode:Auto" ("Type")) -> (x = y?=w209:bool)
            n202 = Greater Than 0?(x=w215) -> (x > 0?=w214:bool)
            n203 = Compound Arithmetic op=OR(w217, w214, w209) -> (w213:bool)
          }
          frame #1 {
            n204 = case shown="True" w220 {
              tunnel: w224 -> [w227 w233]
              tunnel: [w226 w232] -> w223
              tunnel: [w227 w231] -> w222
              tunnel: w221 -> [w226 w229]
              tunnel: w219 -> [_ w228]
              frame False {
                w225 = ""
                n205 = property on="write buffer" class="Str"("Value"=w225) -> ()  [unwired: 2 in, 2 out]
                n206 = property on="read buffer" class="Str"("Value"=w225) -> ()  [unwired: 2 in, 2 out]
              }
              frame True {
                (unwired) u32 6000 ("byte count")
                n207 = VISA Read(VISA resource name=w233, byte count=w228, error in (no error)=w229) -> (VISA resource name out=w231:refnum<visa-resource-name>, read buffer=→"read buffer":string, error out=w232:errorcluster)  [unwired: 1 out]
              }
            }
          }
          frame #2 {
          }
        }
        n208 = Equal?(x=w117, y="Terdeteksi") -> (x = y?=w112:bool)
        n209 = Equal?(x=w132, y=w129) -> (x = y?=w131:bool)
        n210 = Equal?(x=w130, y=w129) -> (x = y?=w128:bool)
        n211 = Get Date/Time In Seconds() -> (seconds since 1Jan1904=w114:timestamp)
        n212 = property on="INFRARED 2" class="Bool (strict)"("Value"=w112) -> ()  [unwired: 2 in, 2 out]
        n213 = Select(t=1, s=w112, f=0) -> (s? t:f=w109:i32)
        n214 = Build Array(w109) -> (w116:i32[])
        n215 = Bundle By Name("Y"=w116, "dt"=1.0, "t0"=w114) -> (→"GRAFIK SENSOR INFRARED":waveform(i32))  [unwired: 1 in]
        n216 = Scan From String(format string="", input string=w136, error in="error in") -> (error out=→"error out 5":errorcluster, output 1=w121:dbl)  [unwired: 2 in, 2 out]
        n217 = property on="POMPA" class="Bool (strict)"("Value"=w131) -> ()  [unwired: 2 in, 2 out]
        n218 = property on="MOTOR 2" class="Bool (strict)"("Value"=w128) -> ()  [unwired: 2 in, 2 out]
        n219 = Get Date/Time In Seconds() -> (seconds since 1Jan1904=w123:timestamp)
        n220 = Build Array(w121) -> (w124:dbl[])
        n221 = property on="WATER LEVEL TANK 2" class="Slide (strict)"("Value"=w121) -> ()  [unwired: 2 in, 2 out]
        n222 = Bundle By Name("Y"=w124, "dt"=1.0, "t0"=w123) -> (→"GRAFIK SENSOR ULTRASONIC":waveform(dbl))  [unwired: 1 in]
        n223 = Greater Or Equal?(x=w121, y=10.0) -> (x >= y?=w118:bool)
        n224 = Less Or Equal?(x=w121, y=3.0) -> (x <= y?=w119:bool)
        n225 = property on="MAX" class="Bool (strict)"("Value"=w118, "Blinking"=w118) -> ()  [unwired: 2 in, 2 out]
        n226 = property on="MIN" class="Bool (strict)"("Value"=w119, "Blinking"=w119) -> ()  [unwired: 2 in, 2 out]
        "Numeric" <- w196
      }
      n227 = call <vilib>:"DB Tools Close Connection.vi"("error in (no error)"=w82, "connection reference"=w78) -> ("error out"=w81:errorcluster)  [unwired: 5 in]
      n228 = VISA Close(VISA resource name=w69, error in (no error)=w70) -> (error out=w80:errorcluster)
      n229 = call <vilib>:"DB Tools Close Connection.vi"("error in (no error)"=w76, "connection reference"=w75) -> ("error out"=w77:errorcluster)  [unwired: 5 in]
      n230 = Merge Errors(w81, w80, w77) -> (→"error out":errorcluster)
    }
  }
  n231 = property on="Combo Box - Autocomplete" class="CmbBox"("Value"=w1) -> ()  [unwired: 2 in, 2 out]
  n232 = property on="Combo Box - Dropdown 2" class="CmbBox"("Value"=w1) -> ()  [unwired: 2 in, 2 out]
  n233 = property on="Login by" class="Str"("Value"=w2) -> ()  [unwired: 2 in, 2 out]
  n234 = property on="Pilihan Sensor & Aktuator" class="CmbBox"("Value"=w2) -> ()  [unwired: 2 in, 2 out]
  n235 = property on="Tab Control" class="TabCtl (strict)"("Value"=enum32{"DashBoard", "Monitoring", "Database"}."DashBoard" ("Tab Control")) -> ()  [unwired: 2 in, 2 out]
